vi "Set_Run_LOG.vi"(0 "列表框 3":refnum<vi>, 1 "组合框":string(combo), 2 "颜色盒":u32(colorbox)=7132, 3 "字符串":string, 5 "error in (no error)":errorcluster caption="错误输入（无错误）") -> (14 "列表框 2":refnum<vi>, 19 "error out":errorcluster caption="错误输出")   [LabVIEW 2018]
panel:
  in  "列表框":i32(listbox)
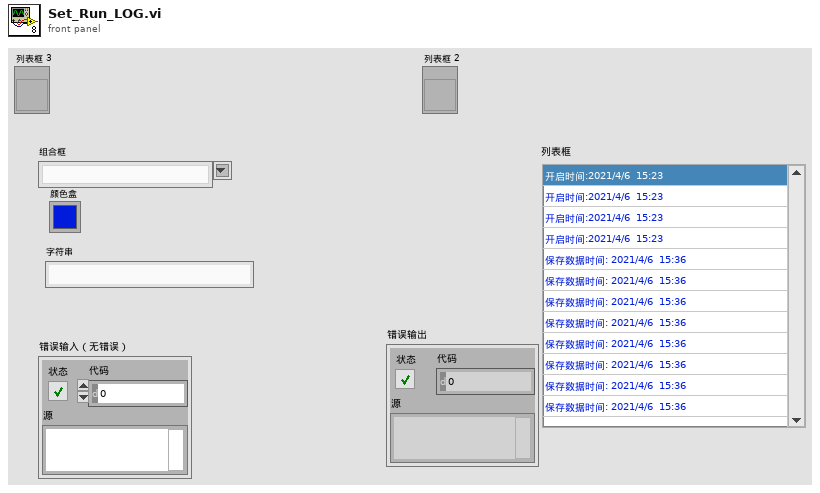
[diagram p1: front panel]
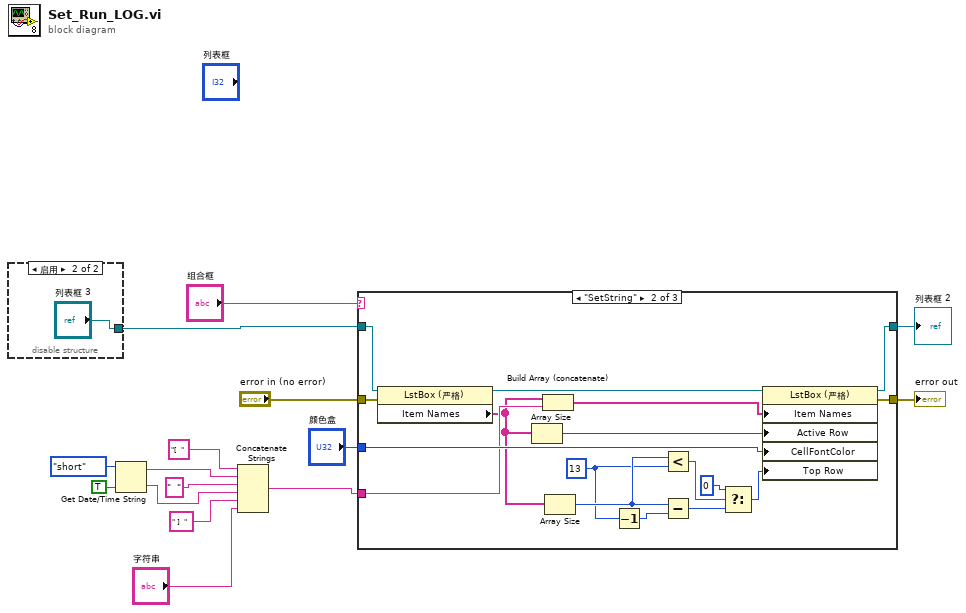
[diagram p0: block diagram]
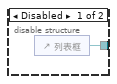
[diagram p2: hidden frame]
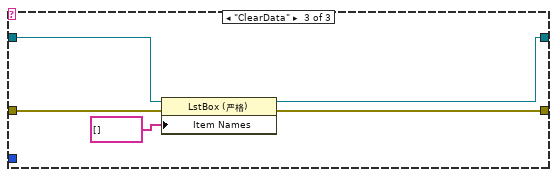
[diagram p4: hidden frame]
diagram:
  n1 = disable-structure shown="启用" {
    disable-tunnel: [w16 "列表框 3"] -> w15
    frame Disabled {
      n2 = control-ref of="列表框"() -> (w16:refnum<vi>)
    }
    frame Enabled {
    }
  }
  n3 = Get Date/Time String(date format (0)=enum16{"short", "long", "abbreviated"}."short" ("日期格式(0)"), want seconds? (F)=TRUE ("需要秒？(F)")) -> (date string=w7:string, time string=w9:string)  [unwired: 1 in]
  n4 = Concatenate Strings("[  ", w7, "  ", w9, " ]  ", "字符串") -> (w4:string)
  n5 = case shown="\"SetString\"" "组合框" {
    tunnel: w15 -> [w19 w36 w40]
    tunnel: "颜色盒" -> [_ w33 _]
    tunnel: w4 -> [_ w32 _]
    tunnel: [w19 w31 w39] -> w10
    tunnel: "error in (no error)" -> [w18 w30 w38]
    tunnel: [w18 w29 w37] -> w11
    frame "假", Default {
    }
    frame "SetString" {
      w20 = 13 ("y")
      n6 = property class="LstBox (严格)"(reference=w36, error in=w30) -> (reference out=w35:refnum<vi>, "Item Names"=w22:string[])  [unwired: 1 out]
      n7 = Array Size(array=w22) -> (size(s)=w34:i32)
      n8 = Build Array (concatenate)(w22, w32) -> (w28:string[])
      n9 = Array Size(array=w22) -> (size(s)=w26:i32)
      n10 = Decrement(x=w20) -> (x-1=w21:i32)
      n11 = Less?(x=w26, y=w20) -> (x < y?=w24:bool)
      n12 = Subtract(x=w26, y=w21) -> (x-y=w25:i32)
      n13 = Select(t=0, s=w24, f=w25) -> (s? t:f=w23:i32)
      n14 = property class="LstBox (严格)"(reference=w35, "Item Names"=w28, "Active Row"=w34, "CellFontColor"=w33, "Top Row"=w23) -> (reference out=w31:refnum<vi>, error out=w29:errorcluster)  [unwired: 1 in]
    }
    frame "ClearData" {
      n15 = property class="LstBox (严格)"(reference=w40, error in=w38, "Item Names"=string[] []) -> (reference out=w39:refnum<vi>, error out=w37:errorcluster)
    }
  }
  "列表框 2" <- w10
  "error out" <- w11
